vi "Update_DestDir_For_Main_Dest_Change.vi"(8 "error in (no error)":errorcluster, 11 "AB_DepSourceDist in":refnum<class "AB_DepSourceDist.lvclass">) -> (0 "error out":errorcluster, 3 "AB_DepSourceDist out":refnum<class "AB_DepSourceDist.lvclass">)   [LabVIEW 2020, in "AB_DepSourceDist.lvclass"]
uses:
  <vilib>/AppBuilder/AB_Classes/DepSourceDist/AB_DepSourceDist.lvclass
  <vilib>/AppBuilder/AB_Classes/DepSourceDist/AB_DepSourceDist.lvclass/AB_DepSourceDist.ctl
  <vilib>/AppBuilder/AB_Classes/Deployment/AB_Deployment.lvlib
  e:/builds/penguin/labview/branches/2020/dev/dist/vi.lib/AppBuilder/AB_Classes/SourceDistribution/AB_SourceDistribution.lvclass
  e:/builds/penguin/labview/branches/2020/dev/dist/vi.lib/AppBuilder/AB_Classes/Build/AB_Build.lvclass
  e:/builds/penguin/labview/branches/2020/dev/dist/vi.lib/AppBuilder/AB_Classes/DepSourceDist/AB_DepSourceDist.lvclass
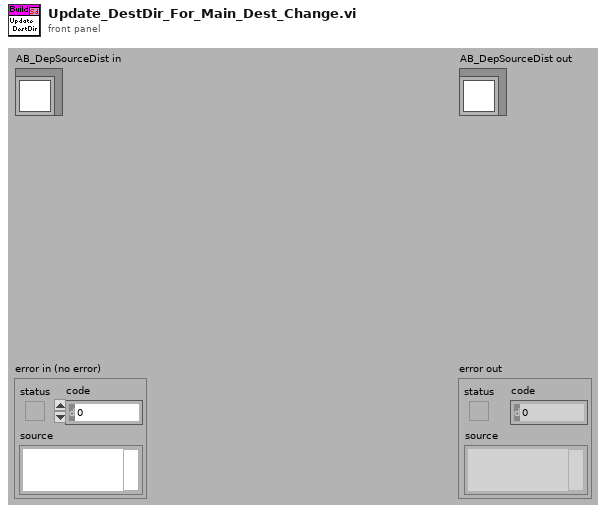
[diagram p1: front panel]
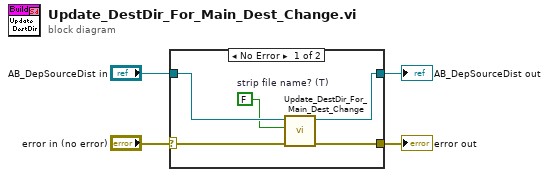
[diagram p0: block diagram]
diagram:
  n1 = case shown="No Error" "error in (no error)" {
    selector: "error in (no error)" -> [w7 w11]
    tunnel: [w6 w11] -> w2
    tunnel: [w8 w10] -> w3
    tunnel: "AB_DepSourceDist in" -> [w9 w10]
    frame No Error {
      w5 = FALSE  # strip file name? (T)
      n2 = call <vilib>:"Update_DestDir_For_Main_Dest_Change.vi"("error in (no error)"=w7, "strip file name? (T)"=w5, "Build in"=w9) -> ("error out"=w6:errorcluster, "Build out"=w8:refnum<class "AB_DepSourceDist.lvclass">)  [unwired: 7 in]
    }
    frame Error {
    }
  }
  "error out" <- w2
  "AB_DepSourceDist out" <- w3
